vi "Set Font.vi"(4 "error in (no error)":errorcluster caption="错误输入（无错误）", 5 "Value":T1 caption="文本字体", 6 "Container State":T3 caption="容器状态", 7 "Display State In":T2={"字符串长度"=10, "过滤字符"=[8, 127], "文本字体"={"Font Name"="", "Size"=0, "Bold"=FALSE, "Italic"=FALSE, "Underline"=FALSE, "Strikeout"=FALSE, "Color"=0}} caption="显示状态输入") -> (0 "error out":errorcluster caption="错误输出", 3 "Display State Out":T2={"字符串长度"=10, "过滤字符"=[8, 127], "文本字体"={"Font Name"="", "Size"=0, "Bold"=FALSE, "Italic"=FALSE, "Underline"=FALSE, "Strikeout"=FALSE, "Color"=0}} caption="显示状态输出")   [LabVIEW 2013, in "Limit String.xctl"]
uses:
  Limit String.xctl
  <vilib>/_xctls/Container State.ctl
  <vilib>/Utility/miscctls.llb/LVFontTypeDef.ctl
  <vilib>/_xctls/XControlSupport.lvlib
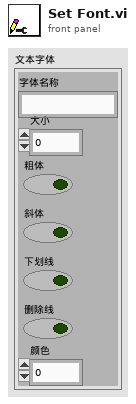
[diagram p1: front panel]
types:
  T1 = typedef "LVFontTypeDef.ctl" = cluster{"Font Name":string, "Size":u16, "Bold":bool, "Italic":bool, "Underline":bool, "Strikeout":bool, "Color":u32}
  T2 = typedef "Limit String.xctl/状态.ctl" = cluster{"字符串长度":u8, "过滤字符":i16[], "文本字体":T1}
  T3 = typedef "XControlSupport.lvlib/Container State.ctl" = cluster{"Indicator?":bool, "Run Mode?":bool, " Refnum":refnum<vi>}
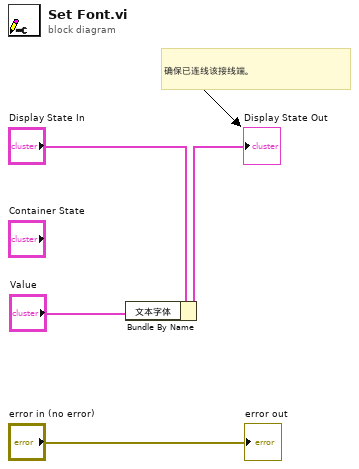
[diagram p0: block diagram]
diagram:
  # "确保已连线该接线端。"
  n1 = Bundle By Name(cluster="Display State In", "文本字体"="Value") -> (→"Display State Out":T2)
  "error out" <- "error in (no error)"
